vi "Cluster Scaling.vi"() -> ()   [LabVIEW 2015]
panel:
  out "Scaled data":T1 {"pressure [N/m^2]" scale=0.0..10.0; "flow rate [liters/sec]" scale=0.0..100.0; "temperature [deg C]" scale=0.0..500.0}
  in  "Raw Data":T2
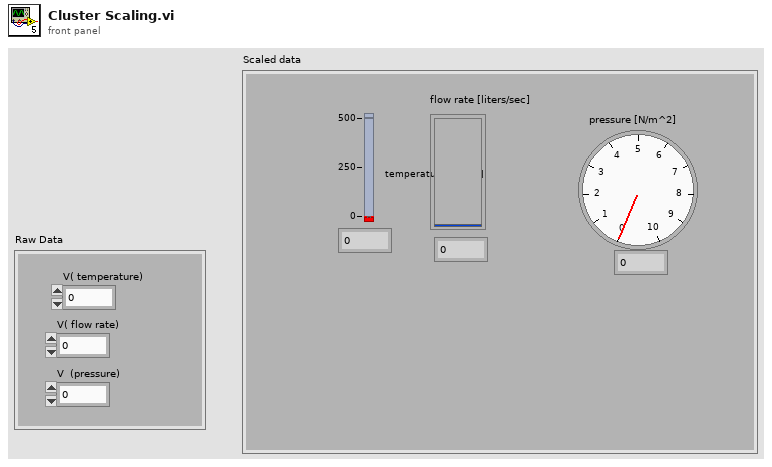
[diagram p1: front panel]
types:
  T1 = cluster{"temperature [deg C]":dbl, "flow rate [liters/sec]":u8, "pressure [N/m^2]":dbl}
  T2 = cluster{"V( temperature)":dbl, "V( flow rate)":dbl, "V  (pressure)":dbl}
  T3 = cluster{"deg C/V":dbl, "(liters/sec)/V":dbl, "(N/m^2)/V":dbl}
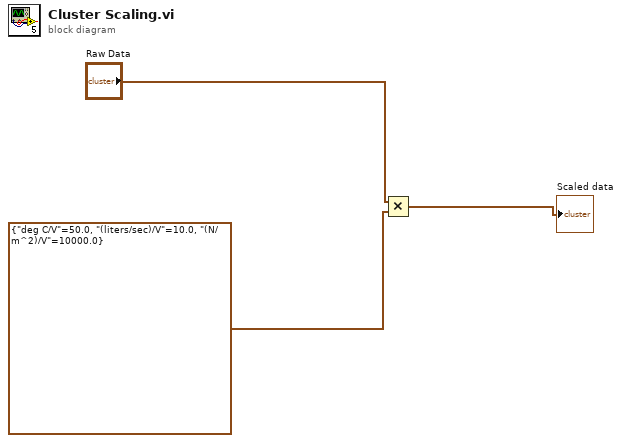
[diagram p0: block diagram]
diagram:
  n1 = Multiply(x="Raw Data", y=T3 {"deg C/V"=50.0, "(liters/sec)/V"=10.0, "(N/m^2)/V"=10000.0}) -> (x*y=→"Scaled data":cluster{dbl, dbl, dbl})
